vi "Build VI Tester Project Provider.vi"() -> ()   [LabVIEW 2017]
panel:
  in  "Remove temp files when finished":bool
  in  "auto-increment version?":bool=TRUE
  in  "Build Project Provider":bool=TRUE
  in  "Package Project Provider":bool
  out "error out":errorcluster
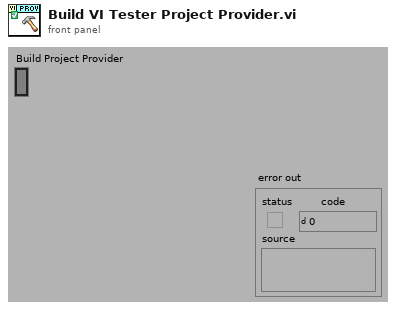
[diagram p1: front panel]
types:
  T1 = enum16{"open", "replace", "create", "open or create", "replace or create", "replace or create with confirmation"}
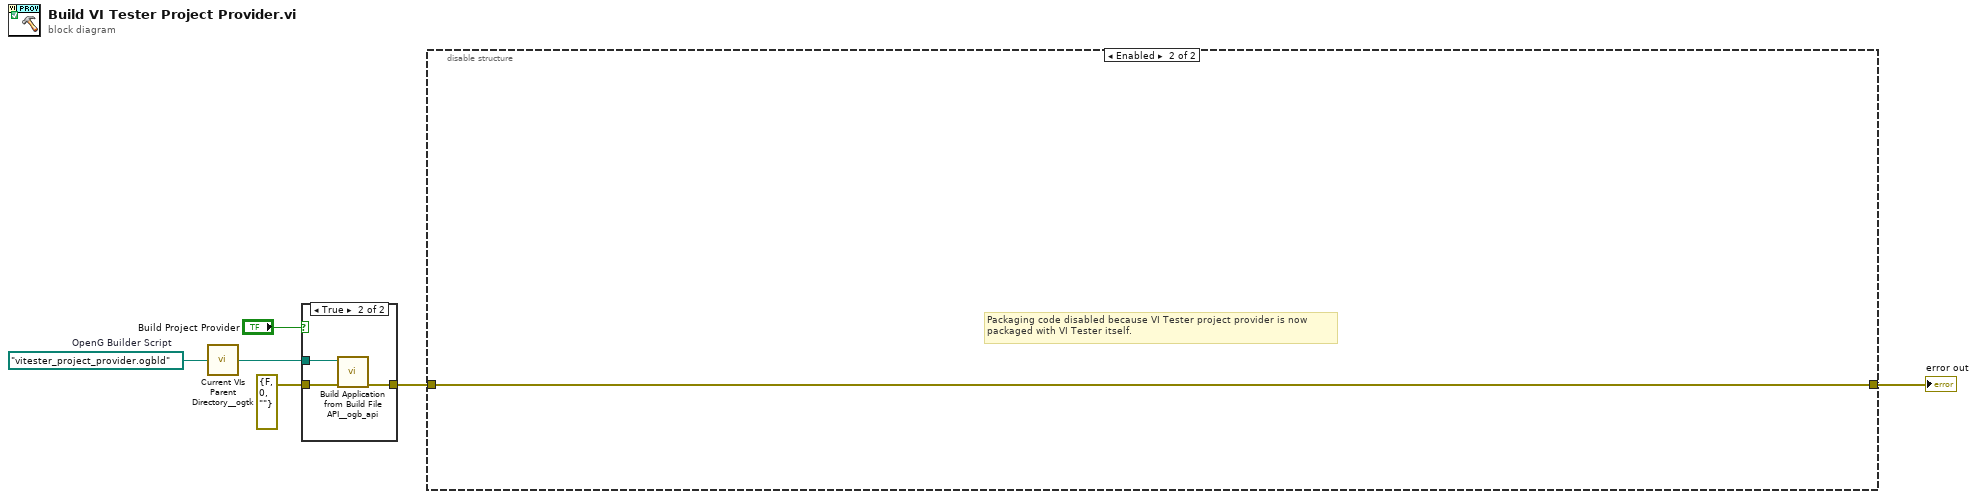
[diagram p0: block diagram]
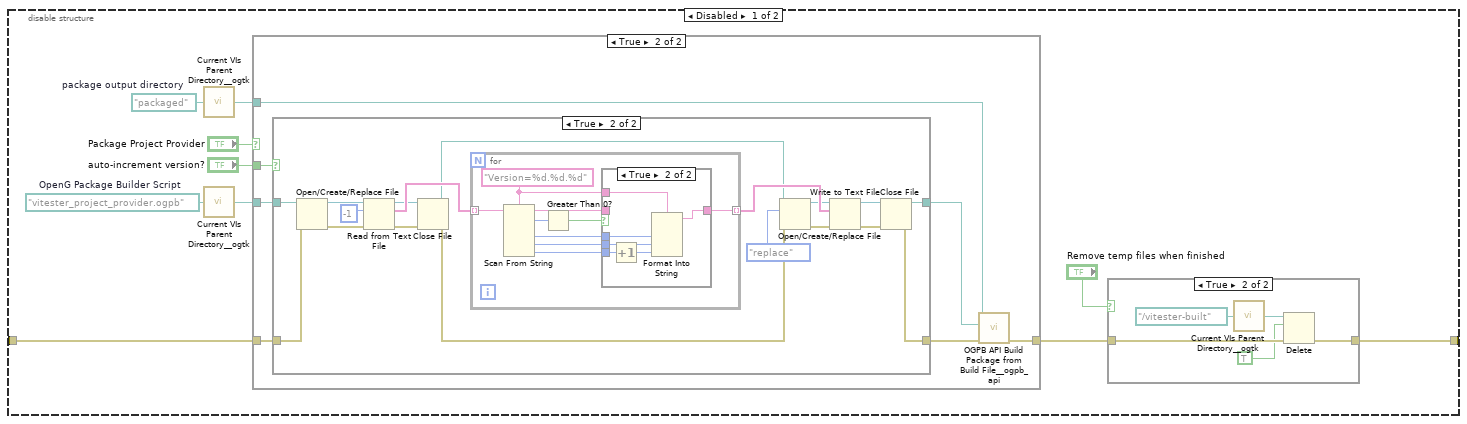
[diagram p2: hidden frame]
diagram:
  w4 = path "vitester_project_provider.ogbld"  # OpenG Builder Script
  n1 = call <userlib>:"Current VIs Parent Directory__ogtk.vi"("Relative path (.)"=w4) -> ("Parent Directory (+ Relative)"=w3:path)  [unwired: 4 in]
  n2 = case shown="True" "Build Project Provider" {
    tunnel: w3 -> [_ w10]
    tunnel: [w7 w9] -> w6
    tunnel: errorcluster {"status"=FALSE, "code"=0, "source"=""} ("error in (no error)") -> [w7 w8]
    frame False {
    }
    frame True {
      n3 = call <userlib>:"Build Application from Build File API__ogb_api.vi"("error in (no error)"=w8, "Build file path"=w10) -> ("error out"=w9:errorcluster)  [unwired: 8 in, 1 out]
    }
  }
  n4 = disable-structure shown="Enabled" {
    disable-tunnel: w6 -> [w20 w71]
    disable-tunnel: [w11 w71] -> w2
    frame Disabled {
      w16 = path "packaged"  # package output directory
      w18 = path "vitester_project_provider.ogpb"  # OpenG Package Builder Script
      n5 = call <userlib>:"Current VIs Parent Directory__ogtk.vi"("Relative path (.)"=w16) -> ("Parent Directory (+ Relative)"=w15:path)  [unwired: 4 in]
      n6 = call <userlib>:"Current VIs Parent Directory__ogtk.vi"("Relative path (.)"=w18) -> ("Parent Directory (+ Relative)"=w17:path)  [unwired: 4 in]
      n7 = case shown="True" "Package Project Provider" {
        tunnel: w20 -> [w27 w32]
        tunnel: [w27 w34] -> w12
        tunnel: w17 -> [_ w30]
        tunnel: w15 -> [_ w33]
        tunnel: "auto-increment version?" -> [_ w28]
        frame False {
        }
        frame True {
          n8 = case shown="True" w28 {
            tunnel: w30 -> [w36 w49]
            tunnel: w32 -> [w35 w47]
            tunnel: [w35 w51] -> w31
            tunnel: [w36 w50] -> w29
            frame False {
            }
            frame True {
              n9 = Open/Create/Replace File(file path (use dialog)=w49, error in=w47) -> (refnum out=w48:refnum<file>, error out=w46:errorcluster)  [unwired: 4 in, 1 out]
              n10 = Read from Text File(file (use dialog)=w48, count=-1, error in=w46) -> (refnum out=w44:refnum<file>, text=w45:string[], error out=w38:errorcluster)  [unwired: 1 in, 1 out]
              n11 = Close File(refnum=w44, error in=w38) -> (path=w42:path, error out=w37:errorcluster)
              n12 = for {
                tunnel: w45 -> [w63] mode=indexing
                tunnel: [w56] -> w43 mode=indexing
                w59 = "Version=%d.%d.%d" ("format string")
                n13 = Scan From String(format string=w59, input string=w63) -> (remaining string=w55:string, offset past scan=w58:u32, output 1=w60:i32, output 2=w61:i32, output 3=w62:i32)  [unwired: 5 in, 1 out]
                n14 = Greater Than 0?(x=w58) -> (x > 0?=w57:bool)
                n15 = case shown="True" w57 {
                  tunnel: w62 -> [_ w70]
                  tunnel: w61 -> [_ w68]
                  tunnel: w60 -> [_ w67]
                  tunnel: w59 -> [_ w66]
                  tunnel: [w64 w65] -> w56
                  tunnel: w55 -> [w64 _]
                  frame False {
                  }
                  frame True {
                    n16 = Increment(x=w70) -> (x+1=w69:i32)
                    n17 = Format Into String(format string=w66, w67, w68, w69) -> (resulting string=w65:string)  [unwired: 2 in, 1 out]
                  }
                }
              }
              n18 = Open/Create/Replace File(file path (use dialog)=w42, error in=w37, operation (0:open)=T1."replace") -> (refnum out=w41:refnum<file>, error out=w39:errorcluster)  [unwired: 3 in, 1 out]
              n19 = Write to Text File(file (use dialog)=w41, text=w43, error in=w39) -> (refnum out=w53:refnum<file>, error out=w52:errorcluster)  [unwired: 1 in, 1 out]
              n20 = Close File(refnum=w53, error in=w52) -> (path=w50:path, error out=w51:errorcluster)
            }
          }
          n21 = call <userlib>:"OGPB API Build Package from Build File__ogpb_api.vi"("error in (no error)"=w31, "Build File path"=w29, "Package Dest Dir"=w33) -> ("error out"=w34:errorcluster)  [unwired: 7 in, 1 out]
        }
      }
      n22 = case shown="True" "Remove temp files when finished" {
        tunnel: w12 -> [w21 w24]
        tunnel: [w21 w23] -> w11
        frame False {
        }
        frame True {
          n23 = call <userlib>:"Current VIs Parent Directory__ogtk.vi"("Relative path (.)"=path "../vitester-built") -> ("Parent Directory (+ Relative)"=w25:path)  [unwired: 4 in]
          n24 = Delete(path (use dialog)=w25, entire hierarchy (F)=TRUE, error in=w24) -> (error out=w23:errorcluster)  [unwired: 2 in, 2 out]
        }
      }
    }
    frame Enabled {
      # "Packaging code disabled because VI Tester project provider is now\npackaged with VI Tester itself."
    }
  }
  "error out" <- w2
